vi "PAN_FindCmdSet3.vi"(6 "defcmdset":string="NATIVE", 10 "cmd in":string) -> (0 "error resp out":errorcluster, 1 "error cmd out":errorcluster, 2 "native cmd out":string, 5 "resp reference":refnum<vi>, 7 "cmdout":string)   [LabVIEW 2016]
panel:
  out "*(type *) &x":u32
  in  "type specifier VI Refnum (for type only) 2":refnum<vi>
  in  "type specifier VI Refnum (for type only)":refnum<vi>
  out "cmdset":string="single_tcp"
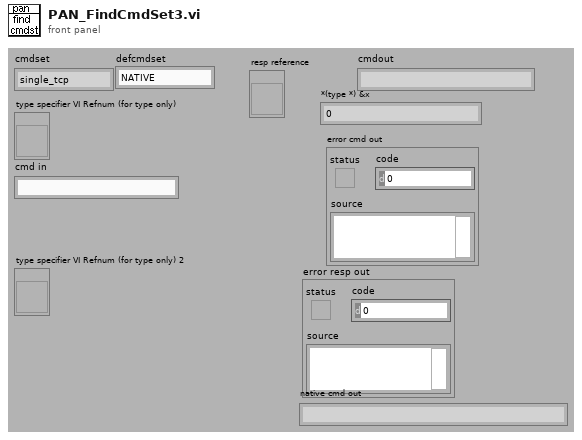
[diagram p1: front panel]
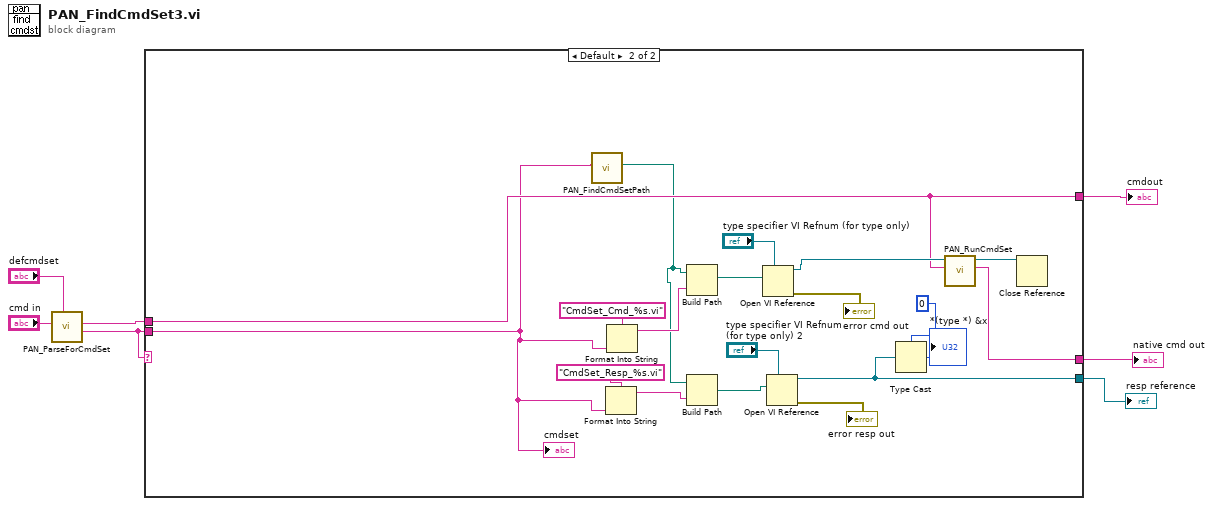
[diagram p0: block diagram]
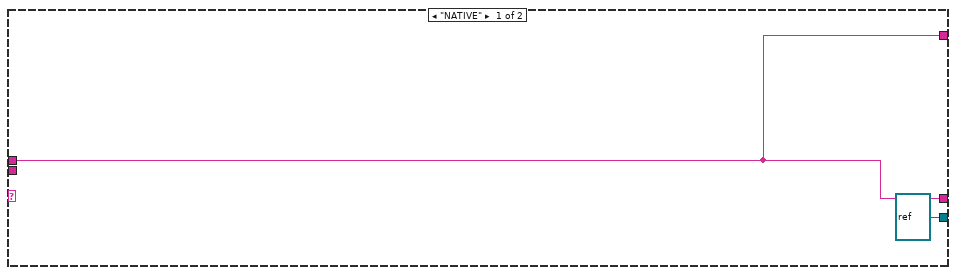
[diagram p2: hidden frame]
diagram:
  n1 = call "PAN_ParseForCmdSet.vi"("defcmdset"="defcmdset", "cmd in"="cmd in") -> ("cmdset"=w2:string, "cmd out"=w6:string)  [unwired: 8 out]
  n2 = case shown="Default" w2 {
    tunnel: w6 -> [w9 w14]
    tunnel: w2 -> [_ w11]
    tunnel: [w9 w14] -> w4
    tunnel: [w9 w13] -> w3
    tunnel: [refnum<vi> refnum ("type specifier VI Refnum (for type only) 2") w12] -> w1
    frame "NATIVE" {
    }
    frame Default {
      n3 = call "PAN_FindCmdSetPath.vi"("cmdset name"=w11) -> ("path"=w10:path)  [unwired: 10 out]
      n4 = Format Into String(format string="CmdSet_Resp_%s.vi", w11) -> (resulting string=w25:string)  [unwired: 2 in, 1 out]
      n5 = Format Into String(format string="CmdSet_Cmd_%s.vi", w11) -> (resulting string=w26:string)  [unwired: 2 in, 1 out]
      n6 = Build Path(base path=w10, name or relative path=w26) -> (appended path=w24:path)
      n7 = Build Path(base path=w10, name or relative path=w25) -> (appended path=w23:path)
      n8 = Open VI Reference(type specifier VI Refnum (for type only)="type specifier VI Refnum (for type only)", vi path=w24) -> (vi reference=w18:refnum<vi>, error out=→"error cmd out":errorcluster)  [unwired: 1 in, 3 out]
      n9 = Open VI Reference(type specifier VI Refnum (for type only)="type specifier VI Refnum (for type only) 2", vi path=w23) -> (vi reference=w12:refnum<vi>, error out=→"error resp out":errorcluster)  [unwired: 1 in, 3 out]
      n10 = Type Cast(type=u32 0, x=w12) -> (*(type *) &x=→"*(type *) &x":u32)
      n11 = call "PAN_RunCmdSet.vi"("cmd in"=w14, "type specifier VI Refnum (for type only)"=w18) -> ("cmd out"=w13:string, "type specifier out"=w15:refnum<vi>)  [unwired: 1 in, 7 out]
      n12 = Close Reference(reference=w15) -> ()  [unwired: 1 in, 1 out]
      "cmdset" <- w11
    }
  }
  "native cmd out" <- w3
  "cmdout" <- w4
  "resp reference" <- w1
